vi "获取扫描电压.vi"(0 "数组":T1[](array[typedef]) {"测试参数"."反向极限电流(mA)" min=0.0 max=3000.0; "测试参数"."反向电压(V)" min=-40.0 max=40.0; "测试参数"."正向极限电流(mA)" min=0.0 max=3000.0; "测试参数"."正向电压(V)" min=-40.0 max=40.0; "时序参数"."反改变量(V)" min=0.0 max=40.0 step=5e-06; "时序参数"."正改变量(V)" min=0.0 max=40.0 step=5e-06; "时序参数"."nplc" min=0.001}) -> (1 "正向扫描电压":dbl[](array[numeric]), 2 "反向扫描电压":dbl[](array[numeric]))   [LabVIEW 2021]
uses:
  2bb48283-cfd2-4234-a952-1209009220c7.vi
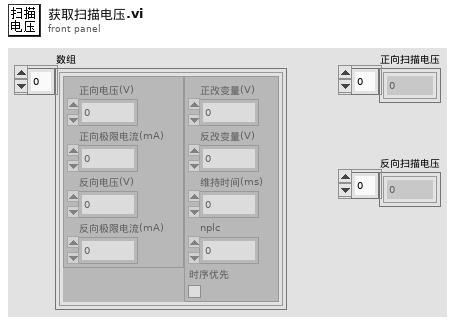
[diagram p1: front panel]
types:
  T1 = typedef "扫描参数.ctl" = cluster{"测试参数":cluster{"正向电压(V)":dbl, "正向极限电流(mA)":dbl, "反向电压(V)":dbl, "反向极限电流(mA)":dbl}, "时序参数":cluster{"正改变量(V)":dbl, "反改变量(V)":dbl, "维持时间(ms)":dbl, "nplc":dbl, "时序优先":bool}}
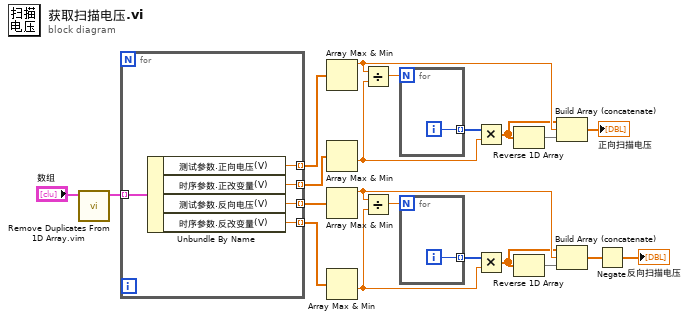
[diagram p0: block diagram]
diagram:
  n1 = call "Remove Duplicates From 1D Array.vim"("array"="数组") -> ("array with duplicates removed"=w2:T1[])  [unwired: 10 in]
  n2 = for {
    tunnel: w2 -> [w26] mode=indexing
    tunnel: [w25] -> w3 mode=indexing
    tunnel: [w22] -> w4 mode=indexing
    tunnel: [w23] -> w5 mode=indexing
    tunnel: [w24] -> w6 mode=indexing
    n3 = Unbundle By Name(w26) -> ("测试参数.正向电压(V)"=w25:dbl, "时序参数.正改变量(V)"=w23:dbl, "测试参数.反向电压(V)"=w22:dbl, "时序参数.反改变量(V)"=w24:dbl)
  }
  n4 = Array Max & Min(array=w3) -> (max value=w18:dbl)  [unwired: 3 out]
  n5 = Array Max & Min(array=w5) -> (min value=w8:dbl)  [unwired: 3 out]
  n6 = Array Max & Min(array=w4) -> (max value=w15:dbl)  [unwired: 3 out]
  n7 = Array Max & Min(array=w6) -> (min value=w10:dbl)  [unwired: 3 out]
  n8 = Divide(x=w18, y=w8) -> (x/y=w11:dbl)
  n9 = Divide(x=w15, y=w10) -> (x/y=w12:dbl)
  n10 = for {
    N: w11 -> [_]
    tunnel: [w27] -> w7 mode=indexing
    i -> [w27]
  }
  n11 = for {
    N: w12 -> [_]
    tunnel: [w28] -> w9 mode=indexing
    i -> [w28]
  }
  n12 = Multiply(x=w7, y=w8) -> (x*y=w17:dbl[])
  n13 = Multiply(x=w9, y=w10) -> (x*y=w13:dbl[])
  n14 = Reverse 1D Array(array=w17) -> (reversed array=w16:dbl[])
  n15 = Reverse 1D Array(array=w13) -> (reversed array=w14:dbl[])
  n16 = Build Array (concatenate)(w17, w18, w16) -> (→"正向扫描电压":dbl[])
  n17 = Build Array (concatenate)(w13, w15, w14) -> (w20:dbl[])
  n18 = Negate(x=w20) -> (-x=→"反向扫描电压":dbl[])
